vi "Untitled 2.vi"() -> ()   [LabVIEW 2023]
uses:
  <vilib>/DAQmx/read.llb/DAQmx Read (Analog Wfm 1Chan NSamp).vi
  <vilib>/DAQmx/configure/timing.llb/DAQmx Timing (Sample Clock).vi
  <vilib>/DAQmx/create/channels.llb/DAQmx Create Channel (AI-Voltage-Basic).vi
  <vilib>/DAQmx/create/channels.llb/DAQmx Create Channel (AO-Voltage-Basic).vi
  <vilib>/DAQmx/configure/timing.llb/DAQmx Timing (Use Waveform).vi
  <vilib>/measure/NI_MABase.lvlib
  <vilib>/DAQmx/configure/trigger.llb/DAQmx Start Trigger (Digital Edge).vi
  <vilib>/DAQmx/write.llb/DAQmx Write (Analog Wfm 1Chan NSamp).vi
panel:
  in  "Settings Button":bool
  in  "Tab Control":enum32{"Page 1", "Page 3", "Page 2"}(tab)
  out "Waveform Chart - Light":dbl(graph)
  out "Image Display":T1(plugin-control)
  out "Waveform Chart":waveform(dbl)(graph)
  in  "Tree":string(tree)
  out "Waveform Graph":waveform(dbl)(graph)
  in  "y":bool
  in  "Cluster":cluster{"#s":dbl, "Fs":dbl}
  in  "stop":bool
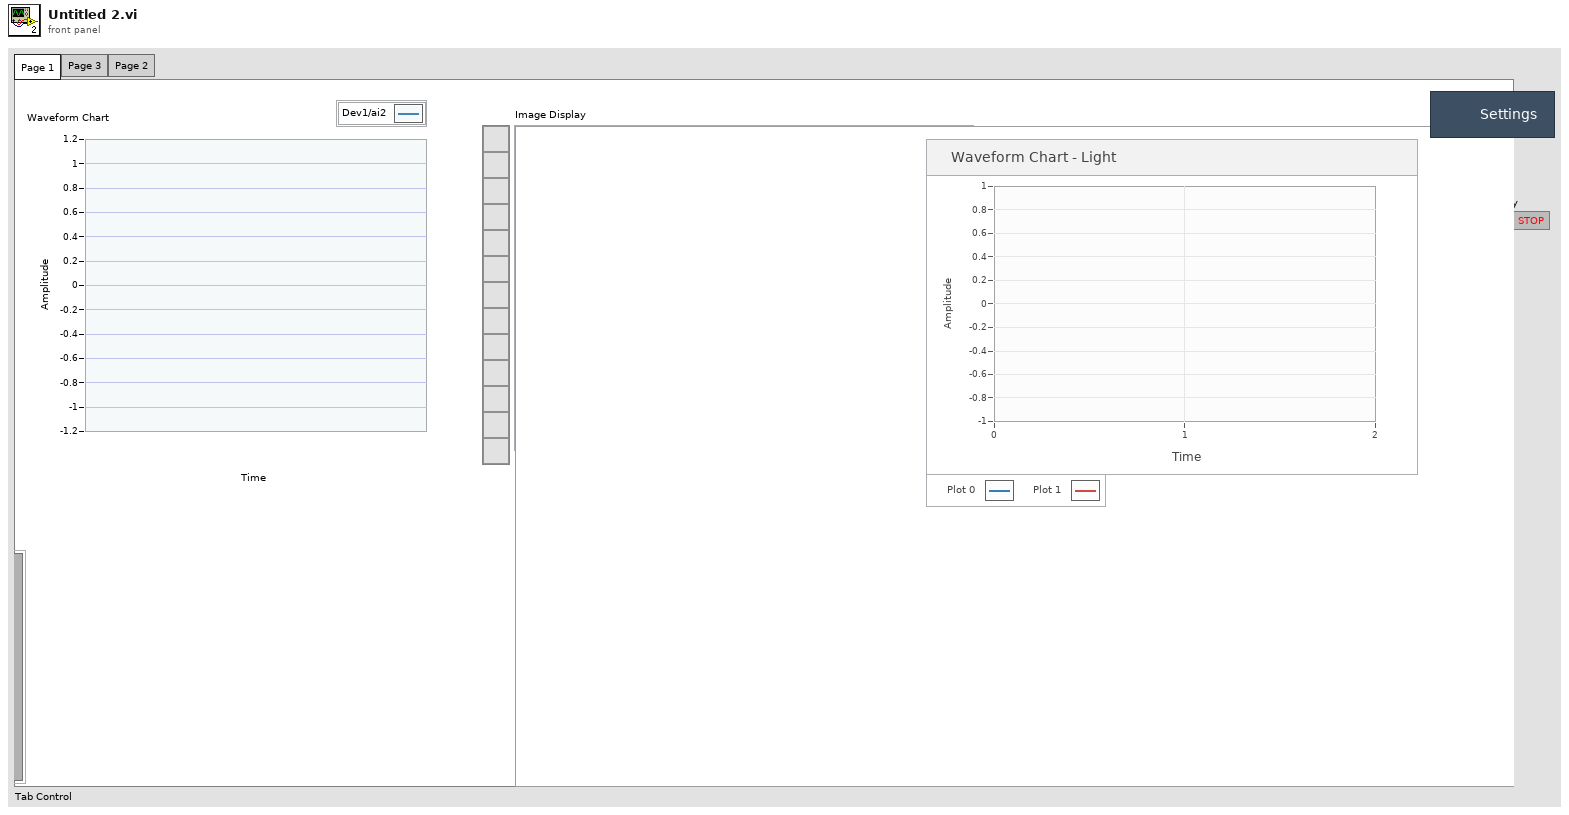
[diagram p1: front panel]
types:
  T1 = typedef "IMAQ Image.ctl" = refnum<image>
  T2 = enum16{"Sine Wave", "Triangle Wave", "Square Wave", "Sawtooth Wave"}
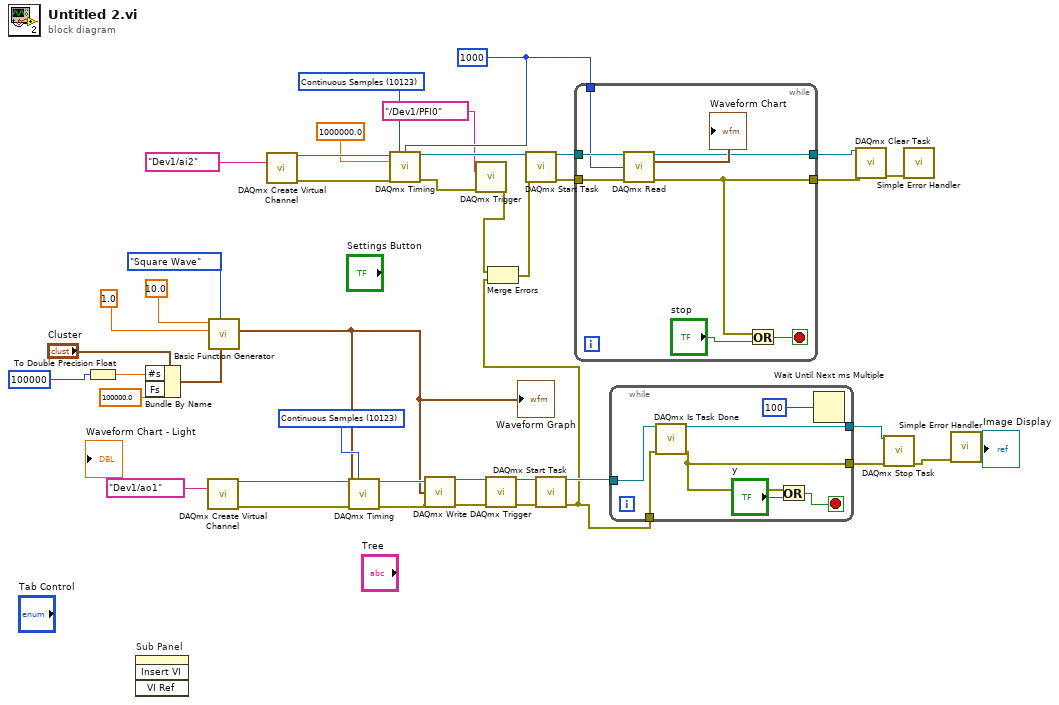
[diagram p0: block diagram]
diagram:
  w23 = 10123 items=["Finite Samples"=10178, "Continuous Samples"=10123, "Hardware Timed Single Point"=12522] ("sample mode")
  w27 = 1000 ("number of samples per channel")
  w28 = 10123 items=["Finite Samples"=10178, "Continuous Samples"=10123, "Hardware Timed Single Point"=12522] ("sample mode")
  n1 = To Double Precision Float(number=100000) -> (double precision float=w16:dbl)
  n2 = invoke on="Sub Panel" class="SubPanel" method="Insert VI"() -> ()  [unwired: 4 in, 4 out]
  n3 = Bundle By Name(cluster="Cluster", "#s"=w16, "Fs"=100000.0) -> (w18:cluster{"#s":dbl, "Fs":dbl})
  n4 = call-poly <vilib>:"DAQmx Create Virtual Channel.vi"("physical channels"=tag "Dev1/ao1") -> ("task out"=w25:refnum<k21>, "error out"=w24:errorcluster)  [unwired: 13 in]
  n5 = call <vilib>:"Basic Function Generator.vi"("sampling info"=w18, "signal type"=T2."Square Wave", "amplitude"=1.0, "frequency"=10.0) -> ("signal out"=w10:waveform(dbl))  [unwired: 5 in, 2 out]
  "Waveform Graph" <- w10
  n6 = call-poly <vilib>:"DAQmx Create Virtual Channel.vi"("physical channels"=tag "Dev1/ai2") -> ("task out"=w37:refnum<k21>, "error out"=w36:errorcluster)  [unwired: 13 in]
  n7 = call-poly <vilib>:"DAQmx Timing.vi"("task/channels in"=w25, "sample mode"=w23, "waveform"=w10, "error in"=w24) -> ("task out"=w14:refnum<k21>, "error out"=w13:errorcluster)  [unwired: 10 in]
  n8 = call-poly <vilib>:"DAQmx Timing.vi"("task/channels in"=w37, "sample mode"=w28, "samples per channel"=w27, "rate"=1000000.0, "error in"=w36) -> ("task out"=w34:refnum<k21>, "error out"=w1:errorcluster)  [unwired: 9 in]
  n9 = call-poly <vilib>:"DAQmx Write.vi"("task/channels in"=w14, "data"=w10, "error in"=w13) -> ("task out"=w9:refnum<k21>, "error out"=w5:errorcluster)  [unwired: 10 in, 1 out]
  n10 = call-poly <vilib>:"DAQmx Trigger.vi"("source"=tag "/Dev1/PFI0", "error in"=w1) -> ("error out"=w2:errorcluster)  [unwired: 12 in, 1 out]
  n11 = call-poly <vilib>:"DAQmx Trigger.vi"() -> ()  [unwired: 14 in, 2 out]
  n12 = call <vilib>:"DAQmx Start Task.vi"("task/channels in"=w9, "error in"=w5) -> ("task out"=w8:refnum<k21>, "error out"=w4:errorcluster)  [unwired: 12 in]
  n13 = Merge Errors(w2, w4) -> (w3:errorcluster)
  n14 = call <vilib>:"DAQmx Start Task.vi"("task/channels in"=w34, "error in"=w3) -> ("task out"=w33:refnum<k21>, "error out"=w32:errorcluster)  [unwired: 12 in]
  n15 = while {
    tunnel: w33 -> [w46]
    tunnel: w32 -> [w45]
    tunnel: [w43] -> w31
    tunnel: [w39] -> w30
    tunnel: w27 -> [w42]
    stop <- w41 stop-if-true
    n16 = call-poly <vilib>:"DAQmx Read.vi"("task/channels in"=w46, "number of samples per channel"=w42, "error in"=w45) -> ("task out"=w43:refnum<k21>, "data"=→"Waveform Chart":waveform(dbl), "error out"=w39:errorcluster)  [unwired: 10 in]
    n17 = Or(x=w39, y="stop") -> (x .or. y?=w41:bool)
  }
  n18 = while {
    tunnel: w8 -> [w53]
    tunnel: w4 -> [w52]
    tunnel: [w49] -> w12
    tunnel: [w48] -> w11
    stop <- w51 stop-if-true
    n19 = call <vilib>:"DAQmx Is Task Done.vi"("task/channels in"=w53, "error in"=w52) -> ("task out"=w49:refnum<k21>, "error out"=w48:errorcluster)  [unwired: 11 in, 1 out]
    n20 = Or(x=w48, y="y") -> (x .or. y?=w51:bool)
    n21 = Wait Until Next ms Multiple(millisecond multiple=u32 100) -> ()  [unwired: 1 out]
  }
  n22 = call <vilib>:"DAQmx Clear Task.vi"("task in"=w31, "error in"=w30) -> ("error out"=w29:errorcluster)  [unwired: 13 in]
  n23 = call <vilib>:"DAQmx Stop Task.vi"("task/channels in"=w12, "error in"=w11) -> ("error out"=w7:errorcluster)  [unwired: 12 in, 1 out]
  n24 = call <vilib>:"Simple Error Handler.vi"("error in (no error)"=w29) -> ()  [unwired: 4 in, 5 out]
  n25 = call <vilib>:"Simple Error Handler.vi"("error in (no error)"=w7) -> ()  [unwired: 4 in, 5 out]
